vi "Init & Start Counter.vi"(8 "error in (no error)":errorcluster, 10 "Config Data":T1={"Auto Refresh"={"Average Mode"=0, "Average Value"=0, "Trigger Mask"=0, "Trigger Mode"=0, "Hardware Trigger Edge"=0, "Hardware Trigger Count"=0, "By Trigger Nbr Of Seq To Acquire"=0, "Time stamp"=FALSE, "Analog Output(mm)"=FALSE, "Invert value"=FALSE, "Temperature value"=FALSE, "Incremental counter value"=FALSE, "Diff. mode"=FALSE}, "Gain"=[], "Offset"=[], "Index"=0, "Range"=0.0, "Sequence"={"Nbr Of Sequence"=0, "Nbr Max Sequence To Transfer"=800, "Delay Mode"=0, "Delay Time Unit"=0, "Delay Value"=0, "Trigger Mask"=5, "Trigger Mode"=0, "Hardware Trigger Edge"=0, "Hardware Trigger Count"=0, "By Trigger Nbr Of Seq To Acquire"=1, "Time stamp"=FALSE, "Sequence counter information"=TRUE, "Analog Output(mm)"=FALSE, "Invert value"=FALSE, "Temperature value"=FALSE, "Incremental counter value"=FALSE, "Diff. mode"=FALSE}, "Enable DIO"=FALSE, "IncCounter"={"CounterMode"="", "CounterOptionDIRECT  "=FALSE, "CounterOptionOthers"=FALSE, "CounterClear "=FALSE, "Cantidad de Pulsos"=0.0, "Reducción"=0.0}, "IncTemperature"={"ConnectedTempSensor"="", "ConvertMode"="", "InitGainSelection"="", "FrequencySelection"="", "PowerSaveMode"=FALSE, "GainSelection"="", "RefValue"=0.0}}, 11 "Connection Data In":T2) -> (0 "error out":errorcluster, 3 "Connection Data Out":T2)   [LabVIEW 2014, in "MSX-E3711_dll.lvlib"]
uses:
  MSX-E3711_dll.lvlib
  Typedef/Connection Data.ctl
  E:/Repositorio Magnis/INF002/v0/Modules/HAL/Drivers/Sync/ADDI-DATA MSX-E3711/API/MSXE371x.dll
  MSXE371x.dll
  E:/Repositorio Magnis/INF002/v0/Modules/HAL/Drivers/Sync/ADDI-DATA MSX-E3711/API/MXCommon.dll
  MXCommon.dll
  Typedef/Config Data.ctl
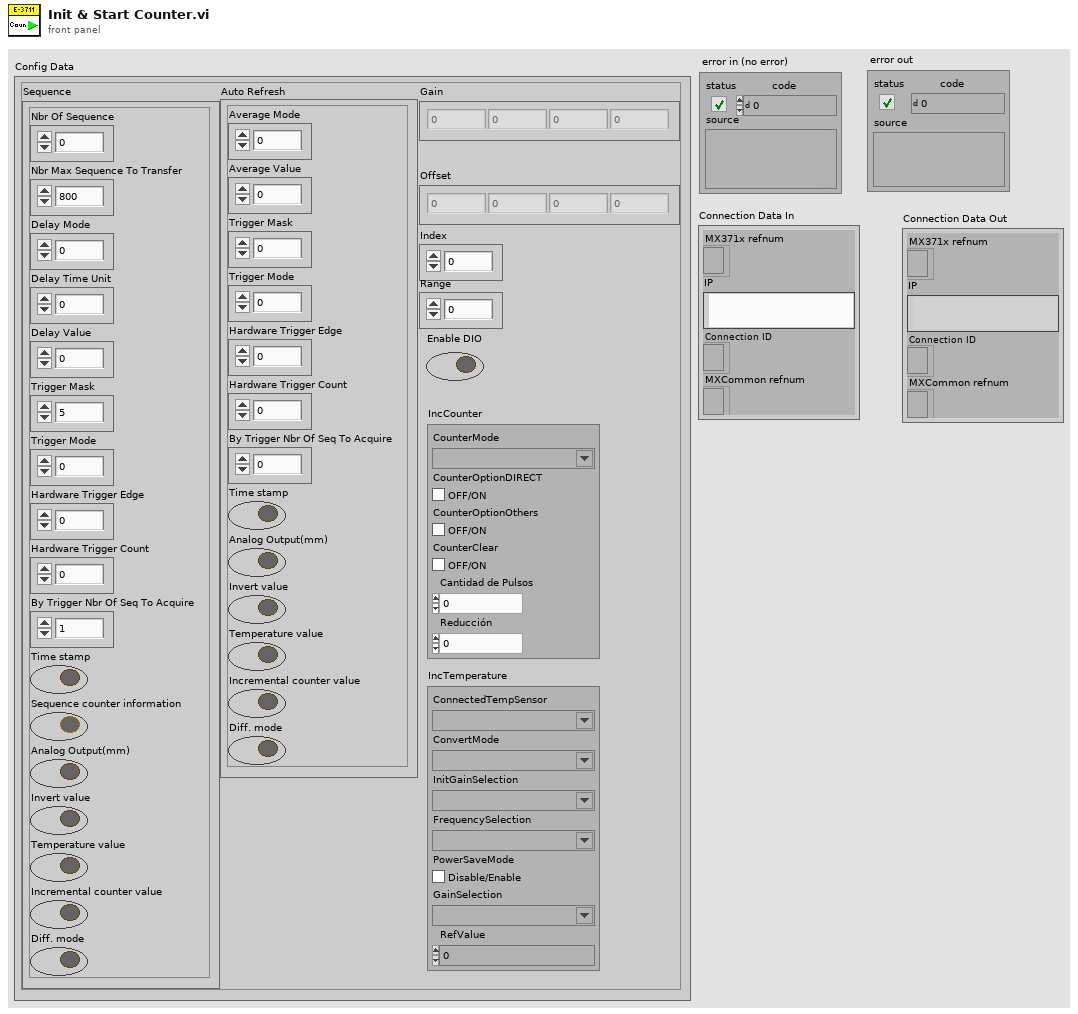
[diagram p1: front panel]
types:
  T1 = typedef "MSX-E3711_dll.lvlib/Config Data.ctl" = cluster{"Auto Refresh":cluster{"Average Mode":u64, "Average Value":u64, "Trigger Mask":u64, "Trigger Mode":u64, "Hardware Trigger Edge":u64, "Hardware Trigger Count":u64, "By Trigger Nbr Of Seq To Acquire":u64, "Time stamp":bool, "Analog Output(mm)":bool, "Invert value":bool, "Temperature value":bool, "Incremental counter value":bool, "Diff. mode":bool}, "Gain":sgl[], "Offset":sgl[], "Index":u64, "Range":sgl, "Sequence":cluster{"Nbr Of Sequence":u64, "Nbr Max Sequence To Transfer":u64, "Delay Mode":u64, "Delay Time Unit":u64, "Delay Value":u64, "Trigger Mask":u64, "Trigger Mode":u64, "Hardware Trigger Edge":u64, "Hardware Trigger Count":u64, "By Trigger Nbr Of Seq To Acquire":u64, "Time stamp":bool, "Sequence counter information":bool, "Analog Output(mm)":bool, "Invert value":bool, "Temperature value":bool, "Incremental counter value":bool, "Diff. mode":bool}, "Enable DIO":bool, "IncCounter":cluster{"CounterMode":string, "CounterOptionDIRECT  ":bool, "CounterOptionOthers":bool, "CounterClear ":bool, "Cantidad de Pulsos":sgl, "Reducción":sgl}, "IncTemperature":cluster{"ConnectedTempSensor":string, "ConvertMode":string, "InitGainSelection":string, "FrequencySelection":string, "PowerSaveMode":bool, "GainSelection":string, "RefValue":dbl}}
  T2 = typedef "MSX-E3711_dll.lvlib/Connection Data.ctl" = cluster{"MX371x refnum":refnum<k24>, "IP":string, "Connection ID ":refnum<k5>, "MXCommon refnum":refnum<k24>}
  T3 = cluster{"CounterMode":string, "CounterOptionDIRECT  ":bool, "CounterOptionOthers":bool, "CounterClear ":bool, "Cantidad de Pulsos":sgl, "Reducción":sgl}
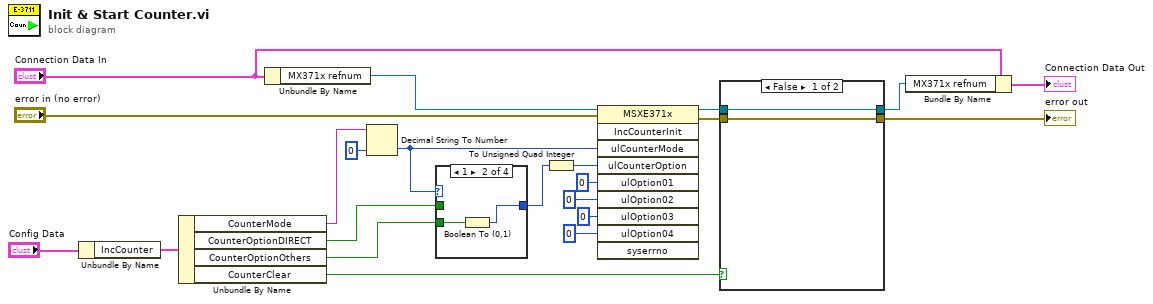
[diagram p0: block diagram]
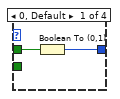
[diagram p2: hidden frame]
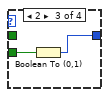
[diagram p3: hidden frame]
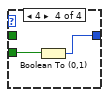
[diagram p4: hidden frame]
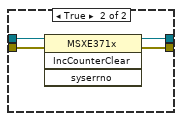
[diagram p5: hidden frame]
diagram:
  n1 = Unbundle By Name("Config Data") -> ("IncCounter"=w17:T3)
  n2 = Unbundle By Name(w17) -> ("CounterMode"=w9:string, "CounterOptionDIRECT"=w6:bool, "CounterOptionOthers"=w5:bool, "CounterClear"=w12:bool)
  n3 = Unbundle By Name("Connection Data In") -> ("MX371x refnum"=w22:refnum<k24>)
  n4 = Decimal String To Number(string=w9, default (0L)=u64 0 ("default (0 I32)")) -> (number=w7:u64)  [unwired: 1 in, 1 out]
  n5 = case shown="1" w7 {
    tunnel: w6 -> [w24 _ _ _]
    tunnel: w5 -> [_ w25 w28 w30]
    tunnel: [w23 w26 w27 w29] -> w3
    frame 0, Default {
      n6 = Boolean To (0,1)(Boolean=w24) -> (0, 1=w23:i16)
    }
    frame 1 {
      n7 = Boolean To (0,1)(Boolean=w25) -> (0, 1=w26:i16)
    }
    frame 2 {
      n8 = Boolean To (0,1)(Boolean=w28) -> (0, 1=w27:i16)
    }
    frame 4 {
      n9 = Boolean To (0,1)(Boolean=w30) -> (0, 1=w29:i16)
    }
  }
  n10 = To Unsigned Quad Integer(1:w3) -> (0:w4:u64)
  n11 = invoke class="MSXE371x" method="IncCounterInit"(reference=w22, error in="error in (no error)", "ulCounterMode"=w7, "ulCounterOption"=w4, "ulOption01"=u64 0, "ulOption02"=u64 0, "ulOption03"=u64 0, "ulOption04"=u64 0) -> (reference out=w10:refnum<k24>, error out=w11:errorcluster)  [unwired: 2 in, 8 out]
  n12 = case shown="False" w12 {
    tunnel: w11 -> [w31 w36]
    tunnel: w10 -> [w32 w35]
    tunnel: [w32 w34] -> w2
    tunnel: [w31 w33] -> w1
    frame False {
    }
    frame True {
      n13 = invoke class="MSXE371x" method="IncCounterClear"(reference=w35, error in=w36) -> (reference out=w34:refnum<k24>, error out=w33:errorcluster)  [unwired: 2 in, 2 out]
    }
  }
  "error out" <- w1
  n14 = Bundle By Name(cluster="Connection Data In", "MX371x refnum"=w2) -> (→"Connection Data Out":T2)
